vi "packing.vi"(8 "error in (no error)":errorcluster, 11 "ColdDrink in":refnum<class "ColdDrink.lvclass">) -> (0 "error out":errorcluster, 2 "Packing.lvclass":refnum<class "Packing.lvclass">, 3 "ColdDrink out":refnum<class "ColdDrink.lvclass">)   [LabVIEW 2017, in "ColdDrink.lvclass"]
uses:
  ColdDrink.lvclass
  Packing Class/Packing.lvclass
  Bottle Class/Bottle.lvclass
  C:/Users/fflores/Documents/LabVIEW-Open-Projects/LabIVEW OOP Design Patterns/Builder Pattern/Packing Class/Packing.lvclass
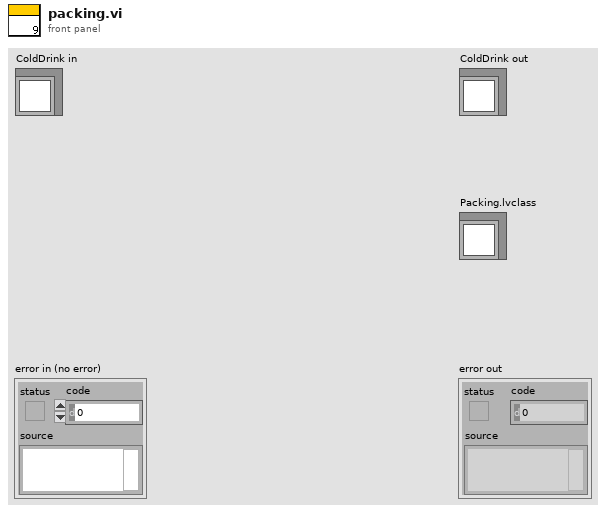
[diagram p1: front panel]
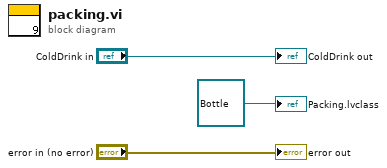
[diagram p0: block diagram]
diagram:
  "error out" <- "error in (no error)"
  "ColdDrink out" <- "ColdDrink in"
  "Packing.lvclass" <- refnum<class "Bottle.lvclass"> refnum ("Bottle.lvclass")
